vi "Write Year.vi"(8 "error in (no error)":errorcluster, 10 "Year":i32, 11 "Vehicle in":refnum<class "Vehicle2.lvclass">) -> (0 "error out":errorcluster, 3 "Vehicle out":refnum<class "Vehicle2.lvclass">)   [LabVIEW 2020, in "ORM_Examples.lvlib" / "Vehicle2.lvclass"]
uses:
  Vehicle2.lvclass
  Vehicle2.lvclass/Vehicle2.ctl
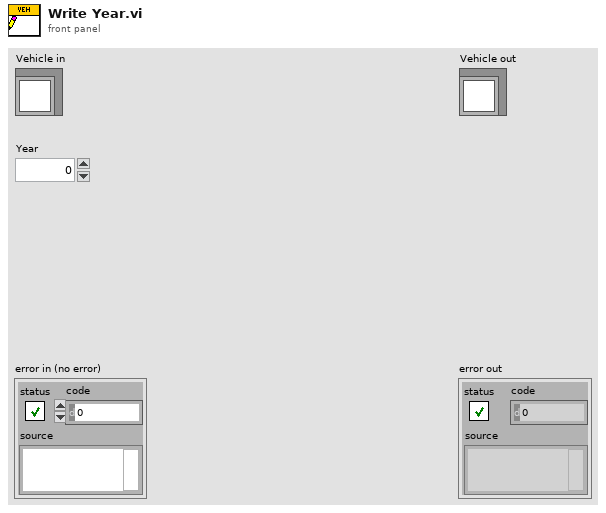
[diagram p1: front panel]
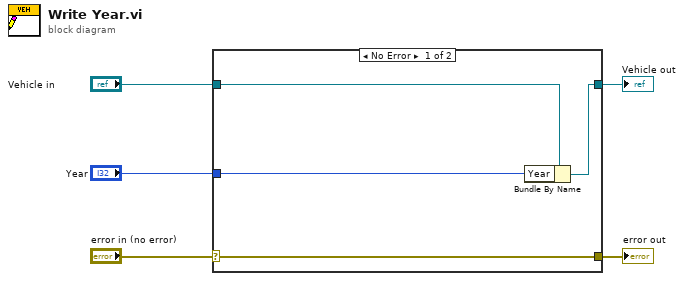
[diagram p0: block diagram]
diagram:
  n1 = case shown="No Error" "error in (no error)" {
    selector: "error in (no error)" -> [w9 w10]
    tunnel: [w9 w10] -> w4
    tunnel: [w7 w11] -> w2
    tunnel: "Vehicle in" -> [w8 w11]
    tunnel: "Year" -> [w6 _]
    frame No Error {
      n2 = Bundle By Name(cluster=w8, "Year"=w6) -> (w7:refnum<class "Vehicle2.lvclass">)
    }
    frame Error {
    }
  }
  "error out" <- w4
  "Vehicle out" <- w2
